vi "Pneumatics_Command_Set_Periodic.vi"(10 "Solenoid Command":T2, 11 "Cluster":T1) -> (3 "Cluster Out":T1)   [LabVIEW 2016]
uses:
  <userlib>/836-libraries/Pneumatics/Support_Code/Pneumatics_Notifier.ctl
  <userlib>/836-libraries/Pneumatics/Support_Code/Pneumatics_Command.ctl
  <userlib>/836-libraries/Pneumatics/Support_Code/Pneumatics_Status.ctl
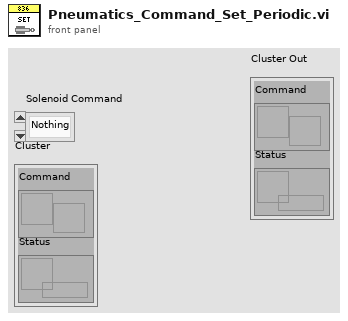
[diagram p1: front panel]
types:
  T1 = typedef "Pneumatics_Notifier.ctl" = cluster{"Command":refnum<notifier>, "Status":refnum<queue>}
  T2 = typedef "Pneumatics_Command.ctl" = enum16{"Nothing", "Forward", "Reverse", "Toggle"}
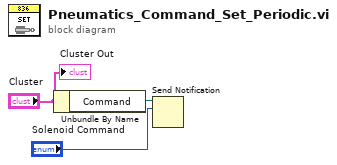
[diagram p0: block diagram]
diagram:
  n1 = Unbundle By Name("Cluster") -> ("Command"=w2:refnum<notifier>)
  n2 = Send Notification(notification="Solenoid Command", notifier=w2) -> ()  [unwired: 1 in, 2 out]
  "Cluster Out" <- "Cluster"
